vi "Grava_ArrayInFile_int.vi"(1 "format (%08x)":string="%08x", 2 "Array to save":u32[](array[numeric]) format="%x", 3 "file name":string, 4 "folder path":path) -> ()   [LabVIEW 2015, in "VIPM2.lvlib"]
doc: "Generic subVI to save an array into a text file, with format %08x.\nTo save: EQ_DATA+Report d'un Chip o Layer; GlobalReg; PixelReg."
uses:
  VIPM2.lvlib
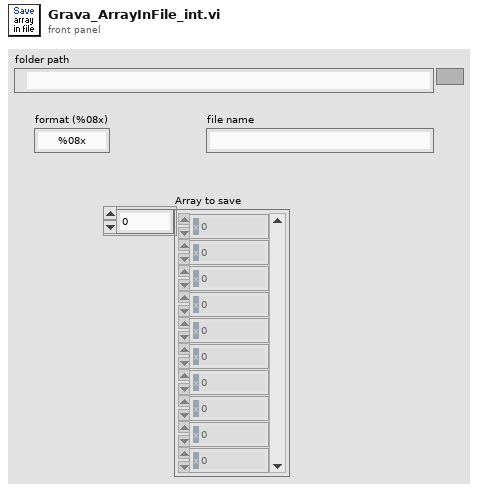
[diagram p1: front panel]
types:
  T1 = enum16{"open", "replace", "create", "open or create", "replace or create", "replace or create with confirmation"}
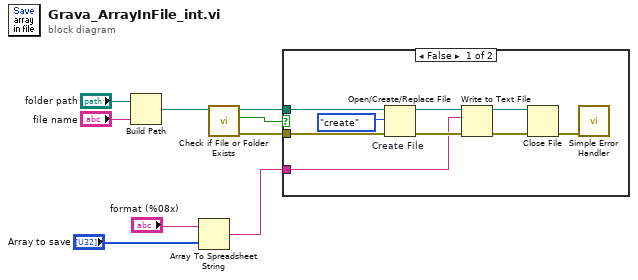
[diagram p0: block diagram]
diagram:
  n1 = Build Path(base path="folder path", name or relative path="file name") -> (appended path=w5:path)
  n2 = Array To Spreadsheet String(array="Array to save", 3:"format (%08x)") -> (spreadsheet string=w2:string)  [unwired: 1 in]
  n3 = call <vilib>:"Check if File or Folder Exists.vi"("path"=w5) -> ("error out"=w4:errorcluster, "file or folder exists?"=w1:bool, "dup path"=w3:path)  [unwired: 8 in]
  n4 = case shown="False" w1 {
    tunnel: w4 -> [w12 _]
    tunnel: w3 -> [w11 _]
    tunnel: w2 -> [w10 _]
    frame False {
      n5 = Open/Create/Replace File "Create File"(file path (use dialog)=w11, error in=w12, operation (0:open)=T1."create") -> (refnum out=w17:refnum<file>, error out=w16:errorcluster)  [unwired: 3 in, 1 out]
      n6 = Write to Text File(file (use dialog)=w17, text=w10, error in=w16) -> (refnum out=w15:refnum<file>, error out=w14:errorcluster)  [unwired: 1 in, 1 out]
      n7 = Close File(refnum=w15, error in=w14) -> (error out=w13:errorcluster)  [unwired: 1 out]
      n8 = call <vilib>:"Simple Error Handler.vi"("error in (no error)"=w13) -> ()  [unwired: 4 in, 5 out]
    }
    frame True {
      # "L'arxiu ja existeix: no el sobreescriguis"
    }
  }
